vi "Out_S2F29.vi"(8 "error in (no error)":errorcluster, 11 "S2 Message Class in":refnum<class "S2 Message Class.lvclass">) -> (0 "error out":errorcluster, 3 "S2 Message Class out":refnum<class "S2 Message Class.lvclass">)   [LabVIEW 2020, in "SECS Communication.lvlib" / "S2 Message Class.lvclass"]
uses:
  S2 Message Class.lvclass
  D:/Dropbox/SECS/SECS_GEM v1.0.6/Com/SECS Communication/SECS-II Class/SECS-II Class.lvclass
  SECS-II Class/Data Message_List.vi
  SECS-II Class/Data Message_U4.vi
  SECS-II Class/SECS-II Class.lvclass
  D:/Dropbox/SECS/SECS_GEM v1.0.6/Com/SECS Communication/S2 Message Class/S2 Message Class.lvclass
panel:
  in  "Equipment Constant ID(ECID)":u32[](array[numeric])
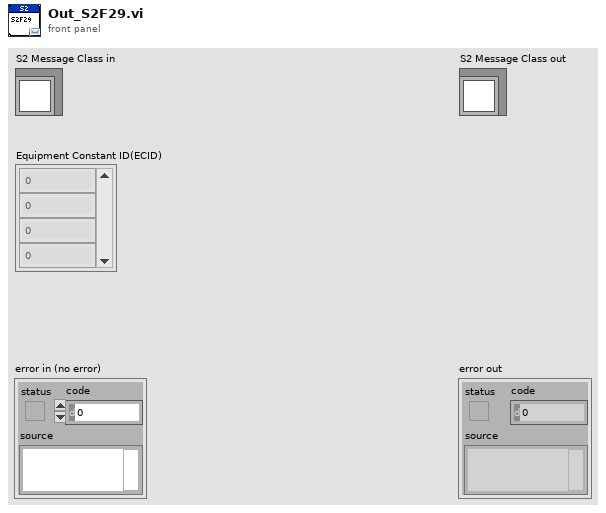
[diagram p1: front panel]
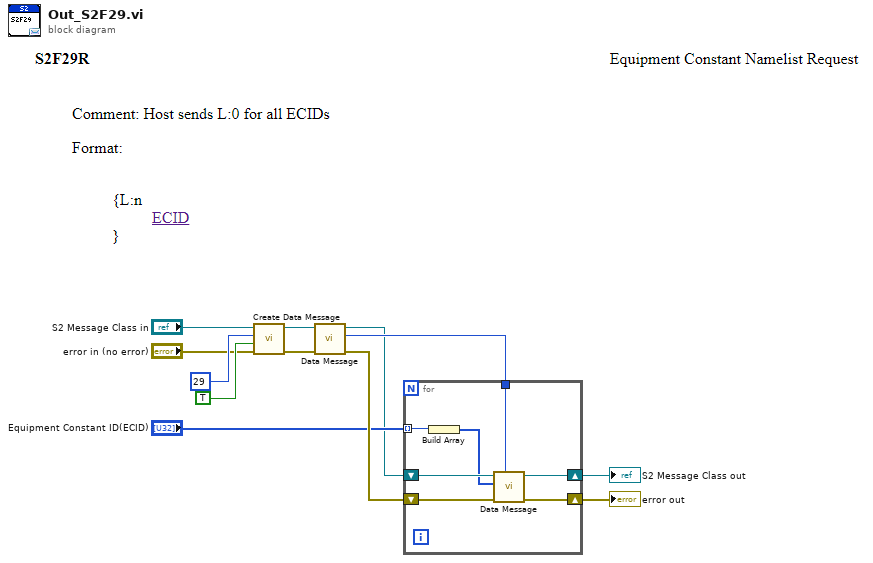
[diagram p0: block diagram]
diagram:
  n1 = call "Create Data Message.vi"("error in (no error)"="error in (no error)", "W-Bit"=TRUE, "Function"=u8 29, "SECS-II Class in"="S2 Message Class in") -> ("error out"=w9:errorcluster, "SECS-II Class out"=w10:refnum<class "S2 Message Class.lvclass">)  [unwired: 6 in]
  n2 = call-poly "Data Message.vi"("error in"=w9, "SECS-II Class in"=w10) -> ("error out"=w5:errorcluster, "Index"=w6:i32, "SECS-II Class out"=w3:refnum<class "S2 Message Class.lvclass">)  [unwired: 7 in]
  n3 = for {
    tunnel: w6 -> [w17]
    shift-right: [w13] -> w1
    shift-left: w5 -> [w18]
    shift-right: [w14] -> w2
    shift-left: w3 -> [w19]
    tunnel: "Equipment Constant ID(ECID)" -> [w16] mode=indexing
    n4 = Build Array(w16) -> (w15:u32[])
    n5 = call-poly "Data Message.vi"("Parent Index"=w17, "error in"=w18, "Data"=w15, "SECS-II Class in"=w19) -> ("error out"=w13:errorcluster, "SECS-II Class out"=w14:refnum<class "S2 Message Class.lvclass">)  [unwired: 6 in]
  }
  "error out" <- w1
  "S2 Message Class out" <- w2
